vi "2_VI_ZED-F9P_GPS-RTK2.vi"(0 "I2C Ref In":T1={"myRIO Reference"={"myRIO Model"=enum."Unknown", "myRIO Hardware Reference"={"Generic FPGA Reference"=refnum, "Allow multiple opens"=FALSE}}, "I2C Channels Enum"=enum."Not Connected", "I2C Configuration"={"I2C Transfer Rate"=enum."Fast mode (400 kbps)"}}, 5 "error in (no error)":errorcluster) -> (14 "output cluster":T9, 19 "error IO":errorcluster)   [LabVIEW 2019]
doc: "VI som omdanner NMEA besked fra GPS-RTK2 board til tid, position og hastighed.\n\nBygget på VI diagram fra dokumentet: \nZED-F9P RTK GPS E2019\nMechatronic challenge group 10\nAarhus University\nThe 21st May 2019"
uses:
  <vilib>/myRIO/Instrument Drivers/Onboard IO/I2C/typedefs/I2C Reference.ctl
  <vilib>/myRIO/Common/Instrument Driver Framework/Utilities/typedefs/myRIO Generic Hardware Reference.ctl
  <vilib>/myRIO/Common/Instrument Driver Framework/Utilities/typedefs/Hardware Version Enum.ctl
  <vilib>/myRIO/Common/Instrument Driver Framework/Utilities/typedefs/myRIO v1.0 Reference.ctl
  <vilib>/myRIO/Common/Instrument Driver Framework/Utilities/typedefs/Generic FPGA Reference.ctl
  <vilib>/myRIO/Common/Instrument Driver Framework/myRIO v1.0/I2C/typedefs/I2C Channels Enum.ctl
  <vilib>/myRIO/Instrument Drivers/Onboard IO/I2C/typedefs/I2C Configuration.ctl
  <vilib>/myRIO/Instrument Drivers/Onboard IO/I2C/typedefs/I2C Transfer Rate.ctl
  <vilib>/Utility/error.llb/Error Cluster From Error Code.vi
  <vilib>/myRIO/Common/Instrument Driver Framework/myRIO v1.0/I2C/vis/myRIO v1.0 Read I2C.vi
  <vilib>/regexp/Match Regular Expression.xnode
  <vilib>/myRIO/Instrument Drivers/Onboard IO/I2C/I2C.lvlib
panel:
  out "error IO 2":errorcluster
  out "Iterations":i32
  out "I2C Ref Out":T1={"myRIO Reference"={"myRIO Model"=enum."Unknown", "myRIO Hardware Reference"={"Generic FPGA Reference"=refnum, "Allow multiple opens"=FALSE}}, "I2C Channels Enum"=enum."Not Connected", "I2C Configuration"={"I2C Transfer Rate"=enum."Fast mode (400 kbps)"}}
  out "Status":string
  out "Longitude":dbl=10.198055833333333
  out "Latitude":dbl=56.17686888888888
  out "Time value":dbl=172057.0
  out "Speed [m/s]":dbl=0.005658888884 format="%#.3g"
  out "GPS signal corruption":bool
  in  "Successive errors allowed":dbl=100.0
  out "Successive errors":dbl=4.0
  out "$GNRMC":string[](array[string])
  in  "milliseconds to wait":u32=150
  in  "Byte Count":u32=600
  # "A = Valid  V = Invalid"
  # "t"
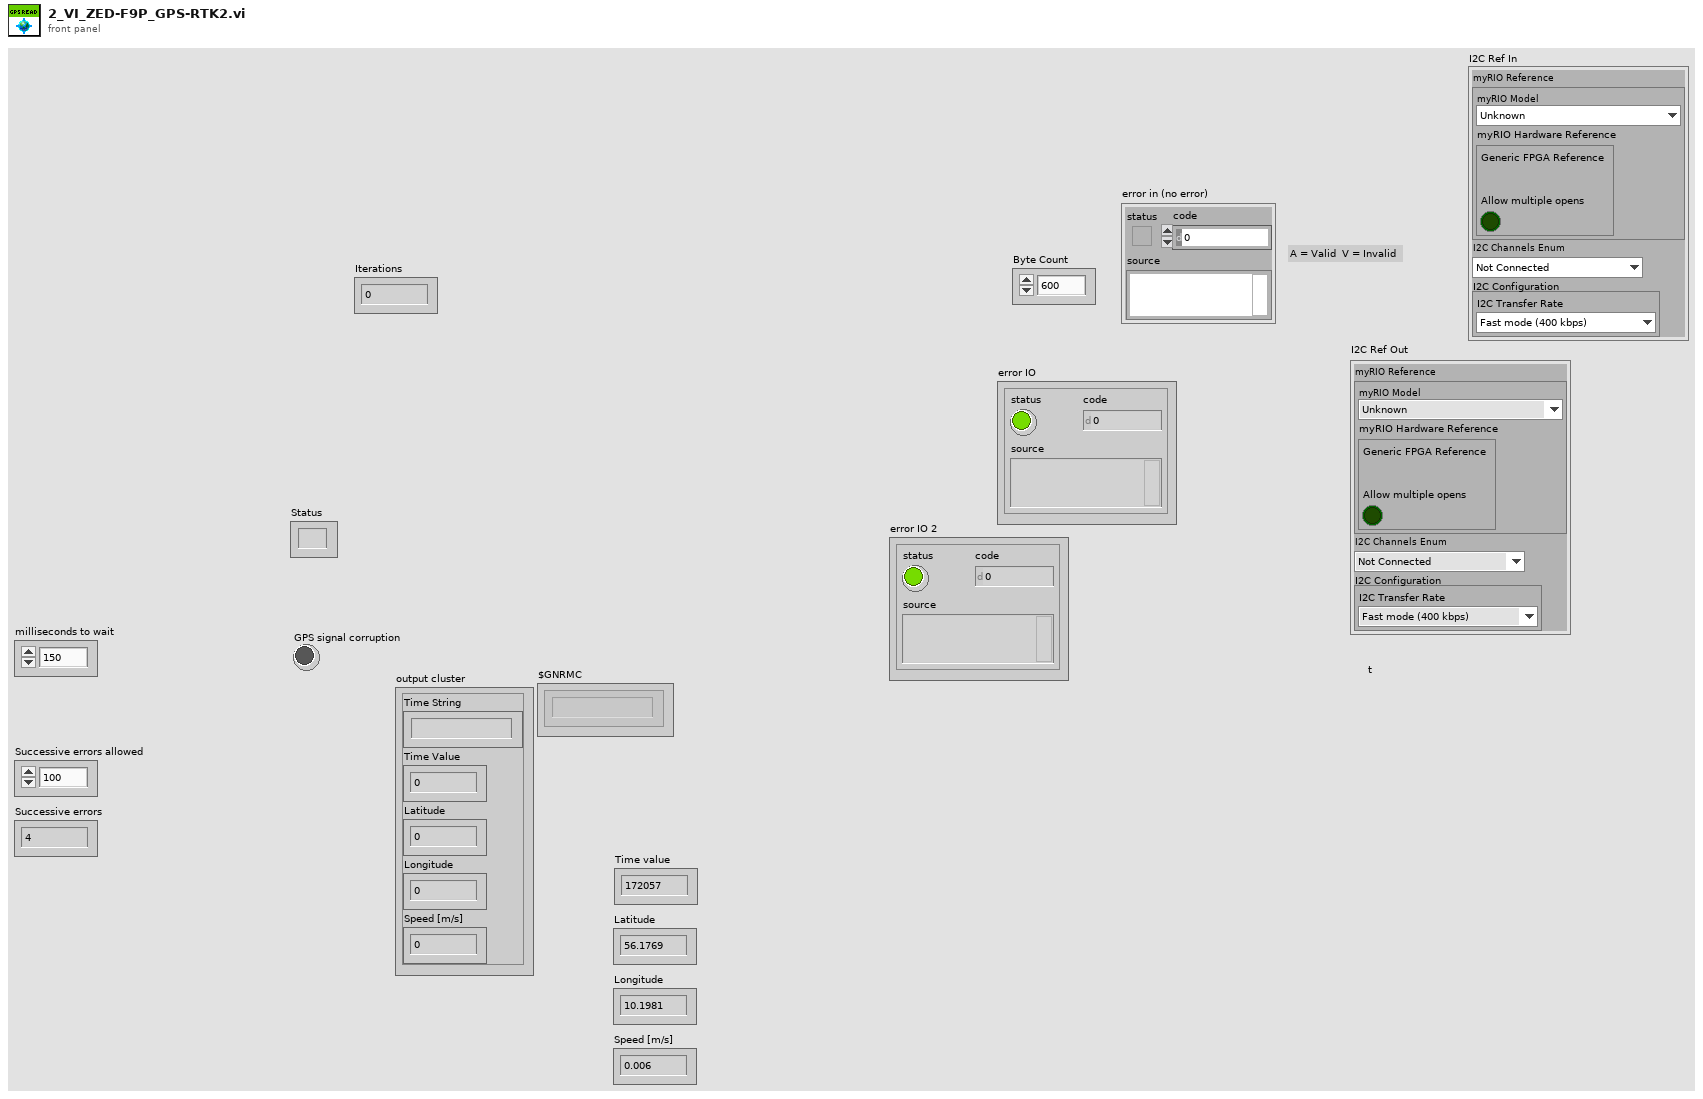
[diagram p1: front panel]
types:
  T1 = typedef "I2C.lvlib/I2C Reference.ctl" = cluster{"myRIO Reference":T2, "I2C Channels Enum":T6, "I2C Configuration":T7}
  T2 = typedef "myRIO Generic Hardware Reference.ctl" = cluster{"myRIO Model":T3, "myRIO Hardware Reference":T4}
  T3 = typedef "Hardware Version Enum.ctl" = enum16{"Unknown", "myRIO-1900", "myRIO-1950", "roboRIO", "NI ELVIS RIO CM", "ELVIS III"}
  T4 = typedef "myRIO v1.0 Reference.ctl" = cluster{"Generic FPGA Reference":T5, "Allow multiple opens":bool}
  T5 = typedef "Generic FPGA Reference.ctl" = refnum<k20>
  T6 = typedef "I2C Channels Enum.ctl" = enum16{"Not Connected", "A/I2C", "B/I2C", "I2C/I2C"}
  T7 = typedef "I2C.lvlib/I2C Configuration.ctl" = cluster{"I2C Transfer Rate":T8}
  T8 = typedef "I2C.lvlib/I2C Transfer Rate.ctl" = enum16{"Standard mode (100 kbps)", "Fast mode (400 kbps)"}
  T9 = cluster{"Time String":string, "Time Value":dbl, "Latitude":dbl, "Longitude":dbl, "Speed [m/s]":dbl}
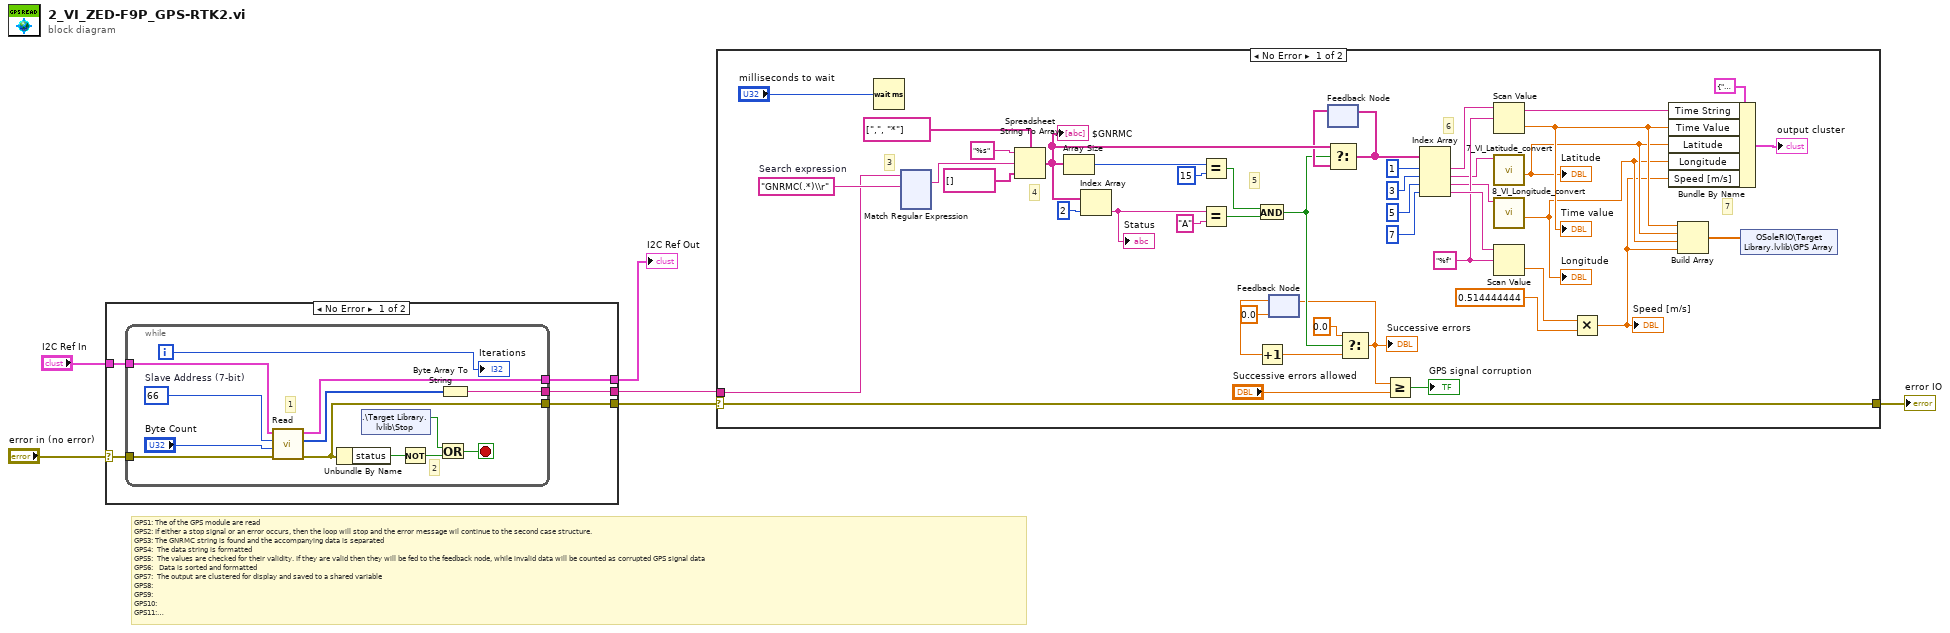
[diagram p0: block diagram]
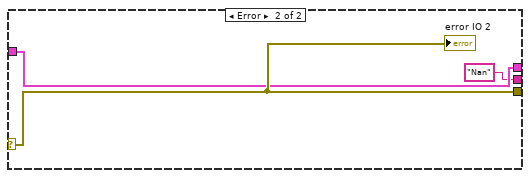
[diagram p2: hidden frame]
diagram:
  # "GPS1: The of the GPS module are read \nGPS2: If either a stop signal or an error occurs, then the loop will stop and the error message wil continue to the second case structure. \nGPS3: The GNRMC string is found and the accompanying data is separated\nGPS4:  The data string is formatted\nGPS5:  The values are checked for their validity. If they are valid then they will be fed to the feedback node, while invalid data will be counted as corrupted GPS signal data\nGPS6:   Data is sorted and formatted\nGPS7:  The output are clustered for display and saved to a shared variable\nGPS8: \nGPS9: \nGPS10: \nGPS11: \nGPS12:"
  n1 = case shown="No Error" "error in (no error)" {
    selector: "error in (no error)" -> [w9 w27]
    tunnel: "I2C Ref In" -> [w11 w26]
    tunnel: [w10 w27] -> w6
    tunnel: [w8 w26] -> w4
    tunnel: [w7 "Nan" ("string")] -> w1
    frame No Error {
      n2 = while {
        tunnel: w11 -> [w24]
        tunnel: [w17] -> w10
        tunnel: w9 -> [w20]
        tunnel: [w16] -> w8
        tunnel: [w15] -> w7
        i -> [w14]
        stop <- w18 stop-if-true
        w22 = u8 66  # Slave Address (7-bit)
        # "2"
        # "1"
        n3 = call <vilib>:"Read.vi"("error in (no error)"=w20, "Byte Count"="Byte Count", "Slave Address (7-bit)"=w22, "I2C Ref In"=w24) -> ("error out"=w17:errorcluster, "Bytes Read"=w21:u8[], "I2C Ref Out"=w16:T1)  [unwired: 4 in]
        n4 = Unbundle By Name(w17) -> ("status"=w13:bool)
        n5 = shared-variable ".\\Target Library.lvlib\\Stop"() -> (w19:bool)  [unwired: 1 in, 1 out]
        n6 = Not(x=w13) -> (.not. x?=w12:bool)
        n7 = Or(x=w19, y=w12) -> (x .or. y?=w18:bool)
        n8 = Byte Array To String(unsigned byte array=w21) -> (string=w15:string)
        "Iterations" <- w14
      }
    }
    frame Error {
      "error IO 2" <- w27
    }
  }
  "I2C Ref Out" <- w4
  n9 = case shown="No Error" w6 {
    selector: w6 -> [w34 w187]
    tunnel: [w34 w187] -> w5
    tunnel: w1 -> [w33 _]
    frame No Error {
      w45 = "%f"
      w71 = "GNRMC(.*)\\r"  # Search expression
      # "7"
      # "6"
      # "5"
      # "4"
      # "3"
      n10 = Wait (ms)(milliseconds to wait="milliseconds to wait") -> ()  [unwired: 1 out]
      n11 = xnode "Match Regular Expression"("input string"=w33, "regular expression"=w71) -> ("whole match"=w70:string)  [unwired: 4 in, 4 out]
      n12 = Spreadsheet String To Array(delimiter (Tab)=string[] [",", "*"], format string="%s", spreadsheet string=w70, array type (2D Dbl)=string[] []) -> (array=w59:string[])
      "$GNRMC" <- w59
      n13 = Array Size(array=w59) -> (size(s)=w65:i32)
      n14 = Index Array(array=w59, index=2) -> (element=w63:string)
      "Status" <- w63
      n15 = Equal?(x=w65, y=15) -> (x = y?=w61:bool)
      n16 = Equal?(x=w63, y="A") -> (x = y?=w60:bool)
      n17 = And(x=w61, y=w60) -> (x .and. y?=w52:bool)
      n18 = feedback #1(0.0 ("t")) -> (w49:dbl)
      n19 = Increment(x=w49) -> (x+1=w50:dbl)
      n20 = feedback #2() -> (w58:string[])  [unwired: 1 in]
      n21 = Select(t=w59, s=w52, f=w58) -> (s? t:f=w57:string[])
      n22 = feedback-in #2(w57) -> ()
      n23 = Select(t=0.0, s=w52, f=w50) -> (s? t:f=w47:dbl)
      "Successive errors" <- w47
      n24 = feedback-in #1(w47) -> ()
      n25 = Greater Or Equal?(x=w47, y="Successive errors allowed") -> (x >= y?=→"GPS signal corruption":bool)
      n26 = Index Array(array=w57, index #1=1 ("index"), index #2=3 ("index"), index #3=5 ("index"), index #4=7 ("index")) -> (element #1=w38:string, element #2=w40:string, element #3=w39:string, element #4=w46:string)
      n27 = Scan Value(string=w38, format string=w45) -> (output string=w36:string, value=w32:dbl)  [unwired: 1 in]
      "Time value" <- w32
      n28 = call "7_VI_Latitude_convert.vi"("Latitude (ddmm.mmmmm)"=w40) -> ("Latitude"=w31:dbl)  [unwired: 9 in]
      "Latitude" <- w31
      n29 = call "8_VI_Longitude_convert.vi"("Longitude (dddmm.mmmmm)"=w39) -> ("Longitude"=w30:dbl)  [unwired: 9 in]
      "Longitude" <- w30
      n30 = Scan Value(string=w46, format string=w45) -> (value=w42:dbl)  [unwired: 1 in, 1 out]
      n31 = Multiply(x=w42, y=0.514444444) -> (x*y=w29:dbl)
      "Speed [m/s]" <- w29
      n32 = Bundle By Name(cluster=T9 {"Time String"="", "Time Value"=0.0, "Latitude"=0.0, "Longitude"=0.0, "Speed [m/s]"=0.0}, "Time String"=w36, "Time Value"=w32, "Latitude"=w31, "Longitude"=w30, "Speed [m/s]"=w29) -> (→"output cluster":T9)
      n33 = Build Array(w32, w31, w30, w29) -> (w28:dbl[])
      n34 = shared-variable "OSoleRIO\\Target Library.lvlib\\GPS Array"(w28) -> ()  [unwired: 1 in, 1 out]
    }
    frame Error {
    }
  }
  "error IO" <- w5
